vi "ConvertdBmtoV.vi"(4 "dBm":dbl) -> (1 "voltage":dbl)   [LabVIEW 2017]
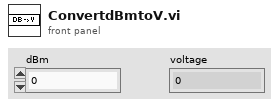
[diagram p1: front panel]
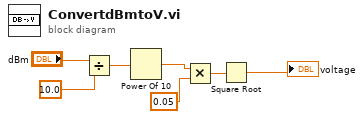
[diagram p0: block diagram]
diagram:
  n1 = Divide(x="dBm", y=10.0) -> (x/y=w5:dbl)
  n2 = Power Of 10(x=w5) -> (10^x=w4:dbl)
  n3 = Multiply(x=w4, y=0.05) -> (x*y=w2:dbl)
  n4 = Square Root(x=w2) -> (sqrt(x)=→"voltage":dbl)
